vi "Main.vi"() -> ()   [LabVIEW 2020]
uses:
  Libraries/Acquisition/Acquisition.lvlib
panel:
  out "Data":dbl[](graph)
  in  "stop":bool
  in  "START":bool
  in  "EXIT":bool
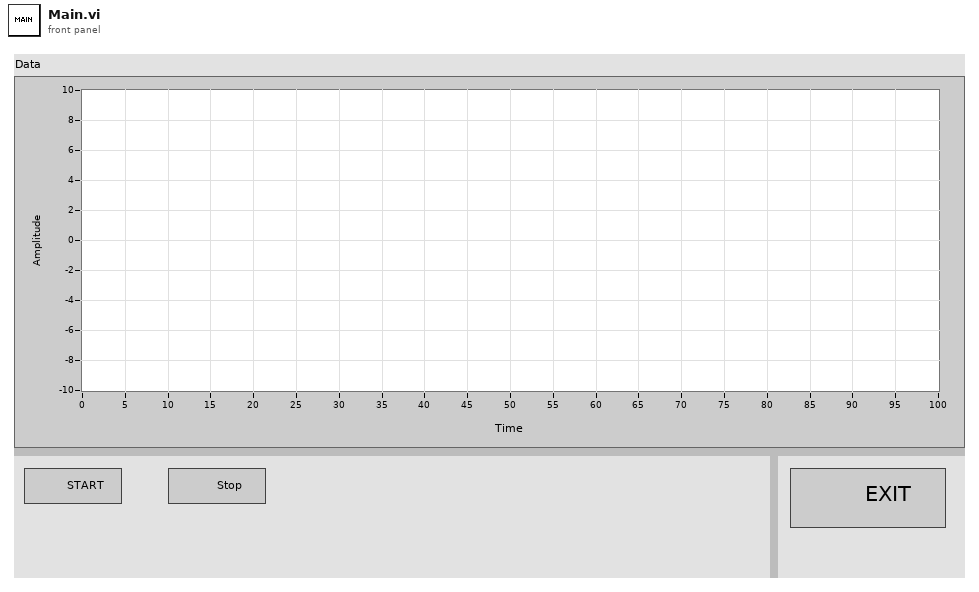
[diagram p1: front panel]
types:
  T1 = typedef "Acquisition.lvlib/Broadcast Events--cluster.ctl" = cluster{"Module Did Init":refnum<user-event>, "Status Updated":refnum<user-event>, "Error Reported":refnum<user-event>, "Module Did Stop":refnum<user-event>, "Update Module Execution Status":refnum<user-event>, "Data Acquired":refnum<user-event>}
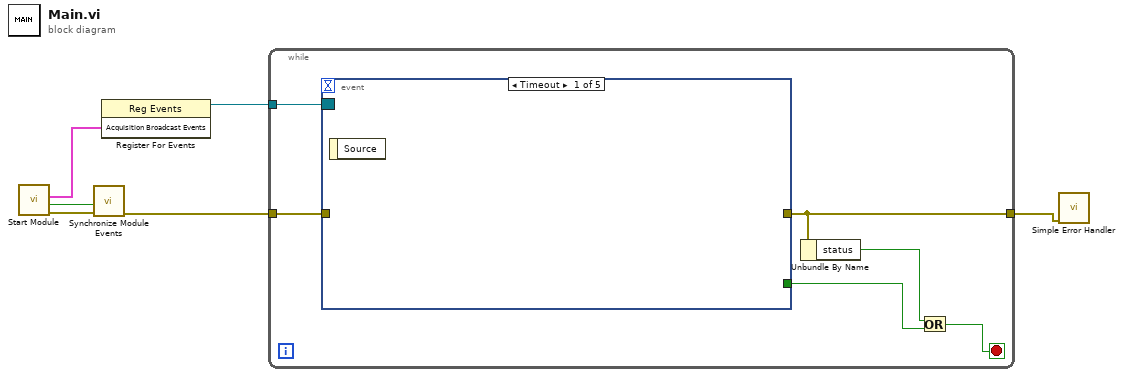
[diagram p0: block diagram]
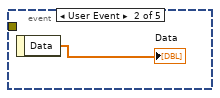
[diagram p2: hidden frame]
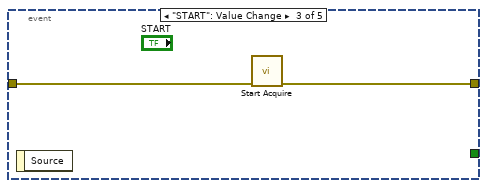
[diagram p3: hidden frame]
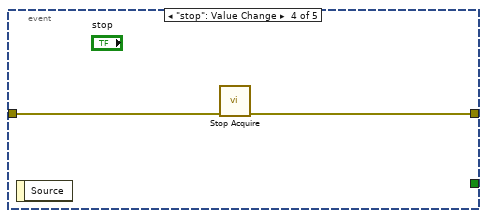
[diagram p4: hidden frame]
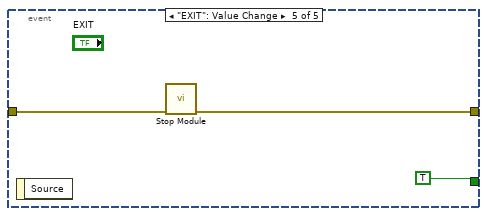
[diagram p5: hidden frame]
diagram:
  n1 = call "Start Module.vi"() -> ("error out"=w6:errorcluster, "Wait for Event Sync?"=w1:bool, "Acquisition Broadcast Events"=w5:T1)  [unwired: 8 in, 1 out]
  n2 = call "Synchronize Module Events.vi"("error in (no error)"=w6, "Wait for Event Sync?"=w1) -> ("error out"=w3:errorcluster)  [unwired: 9 in]
  n3 = register-events(w5) -> (reference out=w4:refnum<event-registration>)  [unwired: 2 in, 1 out]
  n4 = while {
    tunnel: w4 -> [w12]
    tunnel: w3 -> [w11]
    tunnel: [w10] -> w2
    stop <- w9 stop-if-true
    n5 = event shown="[0] Timeout" {
      selector: w12 -> [_ _ _ _ _]
      dyn-events: _ -> [_ _ _ _ _]
      timeout: _ -> [_ _ _ _ _]
      tunnel: w11 -> [_ _ w15 w17 w20]
      tunnel: [_ _ w14 w16 w19] -> w10
      tunnel: [_ _ _ _ TRUE] -> w7
      event Timeout {
        n6 = event-data() -> ()  [unwired: 1 in, 1 out]
      }
      event User Event {
        n7 = event-data() -> ("Data"=→"Data":dbl[])  [unwired: 1 in]
      }
      event "START": Value Change {
        n8 = event-data() -> ()  [unwired: 1 in, 1 out]
        n9 = call "Start Acquire.vi"("error in (no error)"=w15) -> ("error out"=w14:errorcluster)  [unwired: 10 in]
      }
      event "stop": Value Change {
        n10 = event-data() -> ()  [unwired: 1 in, 1 out]
        n11 = call "Stop Acquire.vi"("error in (no error)"=w17) -> ("error out"=w16:errorcluster)  [unwired: 10 in]
      }
      event "EXIT": Value Change {
        n12 = event-data() -> ()  [unwired: 1 in, 1 out]
        n13 = call "Stop Module.vi"("error in (no error)"=w20) -> ("error out"=w19:errorcluster)  [unwired: 10 in]
      }
    }
    n14 = Unbundle By Name(w10) -> ("status"=w8:bool)
    n15 = Or(x=w8, y=w7) -> (x .or. y?=w9:bool)
  }
  n16 = call <vilib>:"Simple Error Handler.vi"("error in (no error)"=w2) -> ()  [unwired: 4 in, 5 out]
